vi "GetOnboardButtons.vi"(11 "packet in":u8[](array[numeric])) -> (3 "onboard buttons state":bool[](array[boolean]))   [LabVIEW 2018]
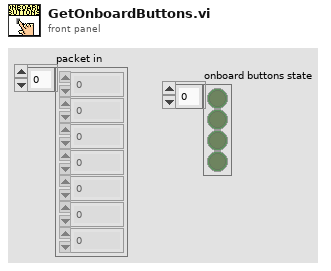
[diagram p1: front panel]
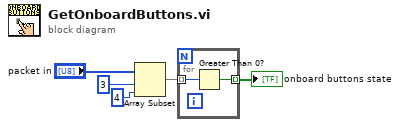
[diagram p0: block diagram]
diagram:
  n1 = Array Subset(array="packet in", index=3, length=4 ("index")) -> (w3:u8[])
  n2 = for {
    tunnel: w3 -> [w7] mode=indexing
    tunnel: [w6] -> w1 mode=indexing
    n3 = Greater Than 0?(x=w7) -> (x > 0?=w6:bool)
  }
  "onboard buttons state" <- w1
